vi "HeatFlow Log Data.vi"(9 "Log Stream":T2, 10 "HeatFlow Res Cfg":T1, 11 "tdms file":refnum<k34>) -> (0 "error out":errorcluster, 2 "Acquisition Stopped?":bool)   [LabVIEW 2019, in "Logging.lvlib"]
doc: "This VI uses the TDMS Write function to write data to a TDMS file."
uses:
  Logging.lvlib
  <extravilib>/ChannelInstances/Stream-var/)Channel.ctl
  HeatFlow Res Cfg.ctl
  HeatFlow Results States.ctl
  Acquisition/HeatFlow/HeatFlow Acq Data.ctl
  <extravilib>/ChannelInstances/Stream-var/Read With Abort.vi
  <extravilib>/ChannelInstances/Stream-var/EndpointRead.vi
  <extravilib>/ChannelInstances/Stream-var/)Channel.vi
  <resource>/ChannelSupport/_ChannelSupport/WaitIfNeeded.vi
  Acquisition/Acquisition.lvlib
  <extravilib>/ChannelInstances/Stream-var.lvlib
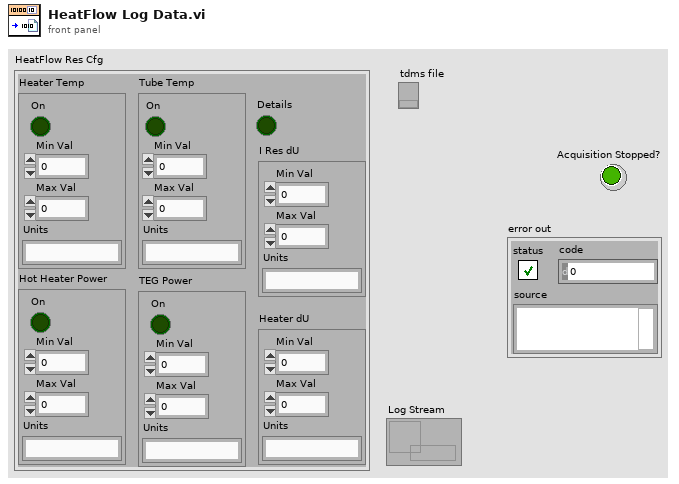
[diagram p1: front panel]
types:
  T1 = typedef "Logging.lvlib/HeatFlow Res Cfg.ctl" = cluster{"Heater Temp":cluster{"On":bool, "Min Val":dbl, "Max Val":dbl, "Units":string}, "Tube Temp":cluster{"On":bool, "Min Val":dbl, "Max Val":dbl, "Units":string}, "Hot Heater Power":cluster{"On":bool, "Min Val":dbl, "Max Val":dbl, "Units":string}, "TEG Power":cluster{"On":bool, "Min Val":dbl, "Max Val":dbl, "Units":string}, "Details":bool, "Heater dU":cluster{"Min Val":dbl, "Max Val":dbl, "Units":string}, "I Res dU":cluster{"Min Val":dbl, "Max Val":dbl, "Units":string}}
  T2 = typedef "Stream-var.lvlib/)Channel.ctl" = refnum<queue>
  T3 = typedef "Acquisition.lvlib/HeatFlow Acq Data.ctl" = cluster{"Time Stamp":timestamp, "Time Delta":u32, "LakeShore_Temp":cluster{"Tube_T_1":dbl, "Tube_T_2":dbl, "Tube_T_3":dbl, "Tube_T_4":dbl, "Tube_T_5":dbl, "Tube_T_6":dbl, "Tube_T_7":dbl, "Tube_T_8":dbl}, "Heaters":cluster{"I_Res_dU":dbl, "Heater_dU":dbl, "Hot_Side_I":dbl, "Hot_Side_P":dbl, "Cold_Ctrl_U":dbl, "Hot_Ctrl_U":dbl, "Hot_Side_T":dbl, "Cold_Side_T":dbl}, "TEG":cluster{"TEG_Load_dU":dbl, "TEG_Load_R":dbl, "TEG_Load_I":dbl, "TEG_Load_P":dbl, "TEG_eta":dbl, "TEG_dT":dbl, "TEG_U_open":dbl, "TEG_U_Test":dbl, "TEG_R_Test":dbl, "TEG_Rw":dbl}, "LastElement?":bool}
  T4 = typedef "Logging.lvlib/HeatFlow Results States.ctl" = enum16{"Start", "Timestamp", "Heater Temp", "Tube Temp", "Heater Power", "TEG Power", "Details", "End"}
  T5 = cluster{"Tube_T_1":dbl, "Tube_T_2":dbl, "Tube_T_3":dbl, "Tube_T_4":dbl, "Tube_T_5":dbl, "Tube_T_6":dbl, "Tube_T_7":dbl, "Tube_T_8":dbl}
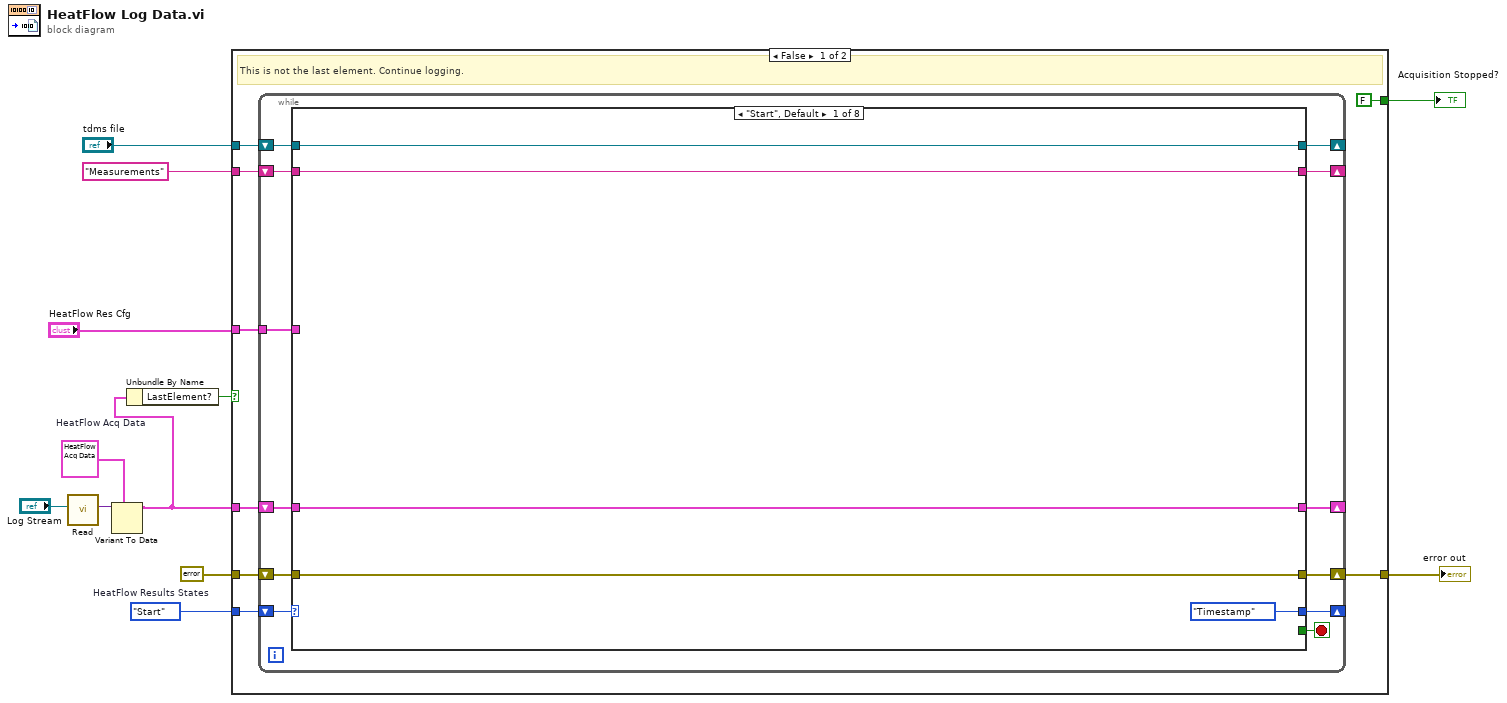
[diagram p0: block diagram]
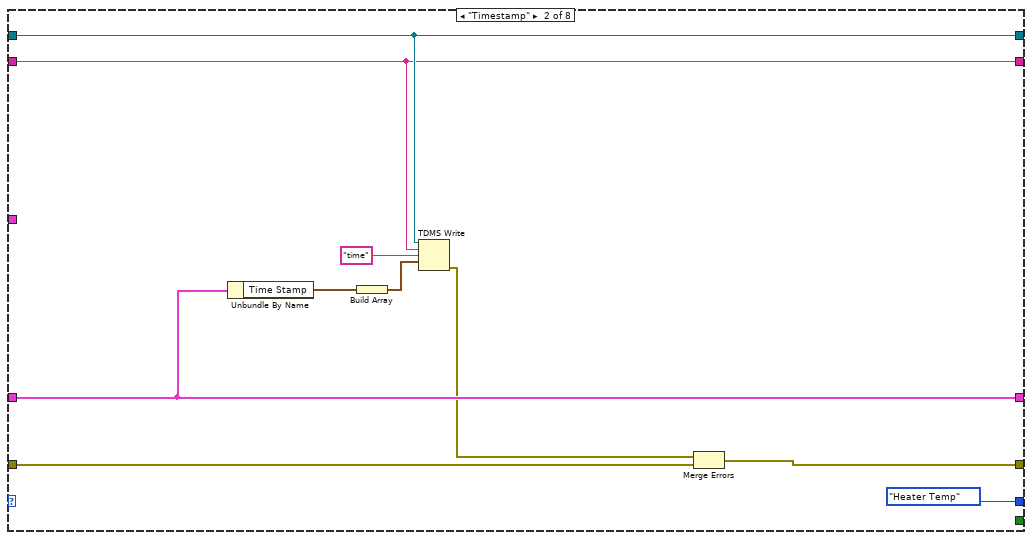
[diagram p2: hidden frame]
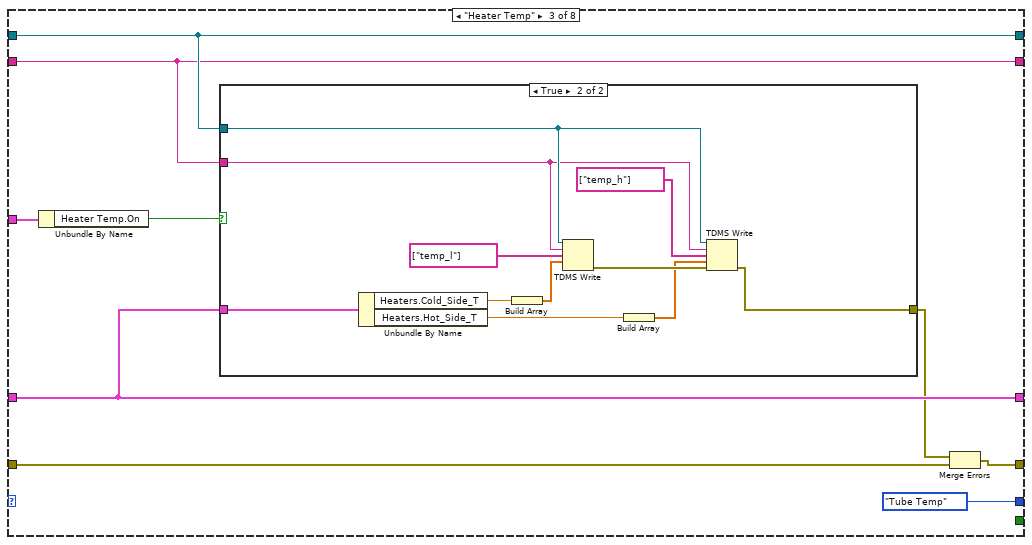
[diagram p3: hidden frame]
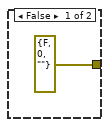
[diagram p4: hidden frame]
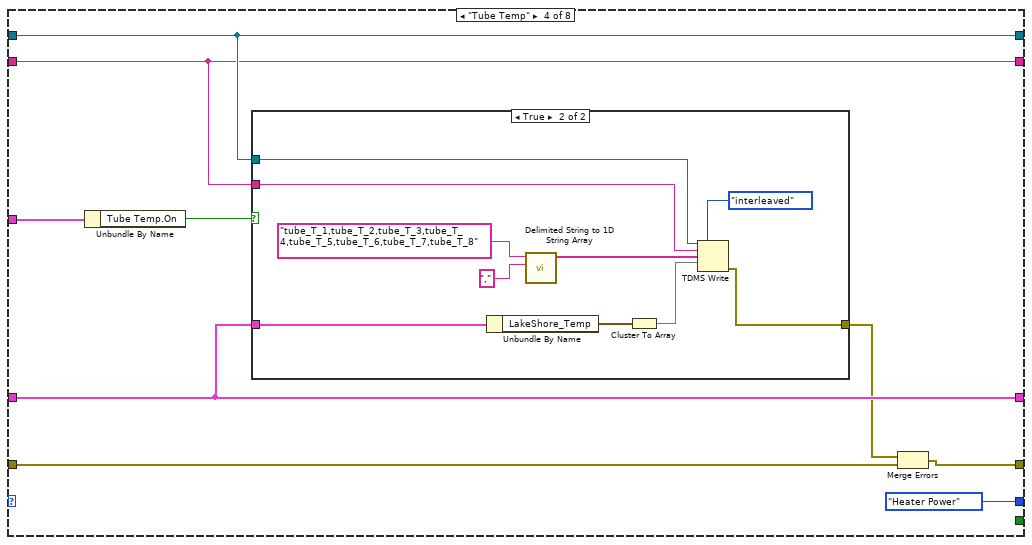
[diagram p5: hidden frame]
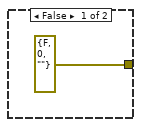
[diagram p6: hidden frame]
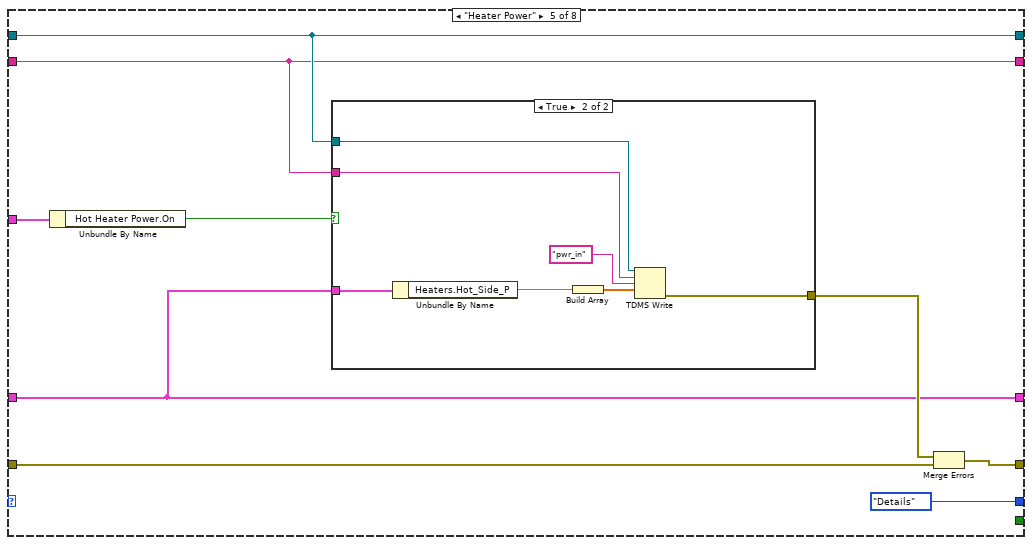
[diagram p7: hidden frame]
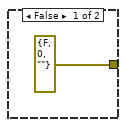
[diagram p8: hidden frame]
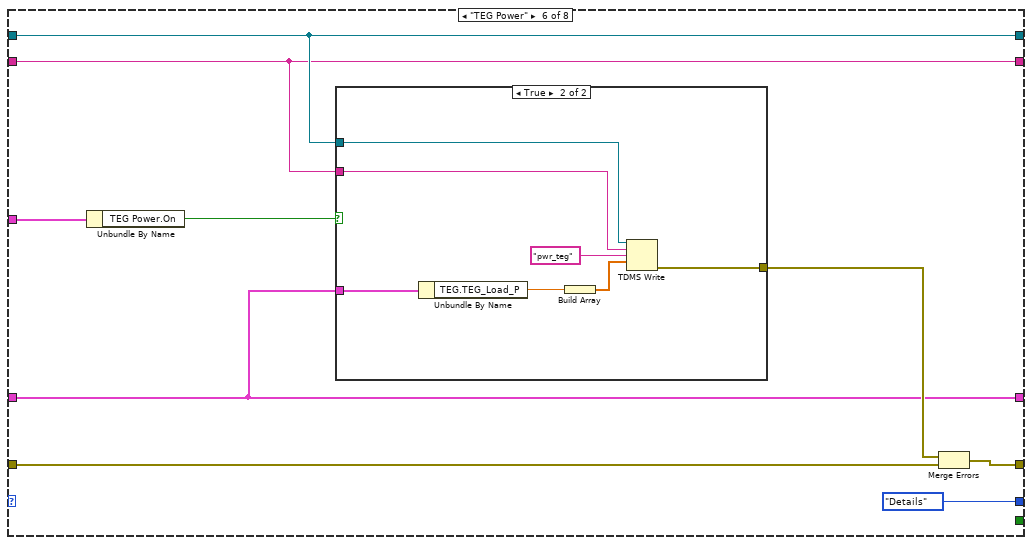
[diagram p9: hidden frame]
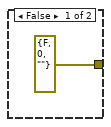
[diagram p10: hidden frame]
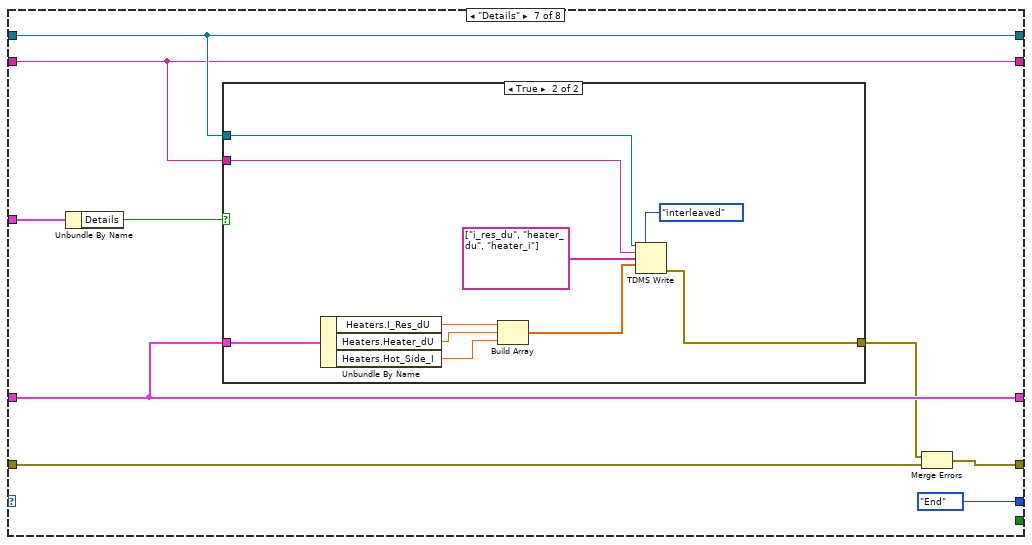
[diagram p11: hidden frame]
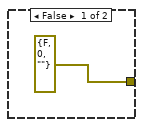
[diagram p12: hidden frame]
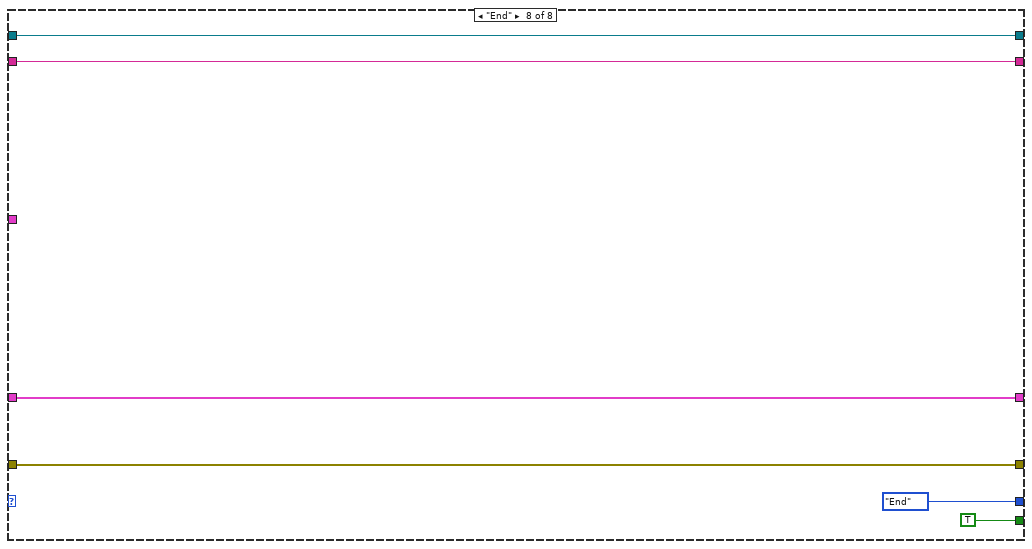
[diagram p13: hidden frame]
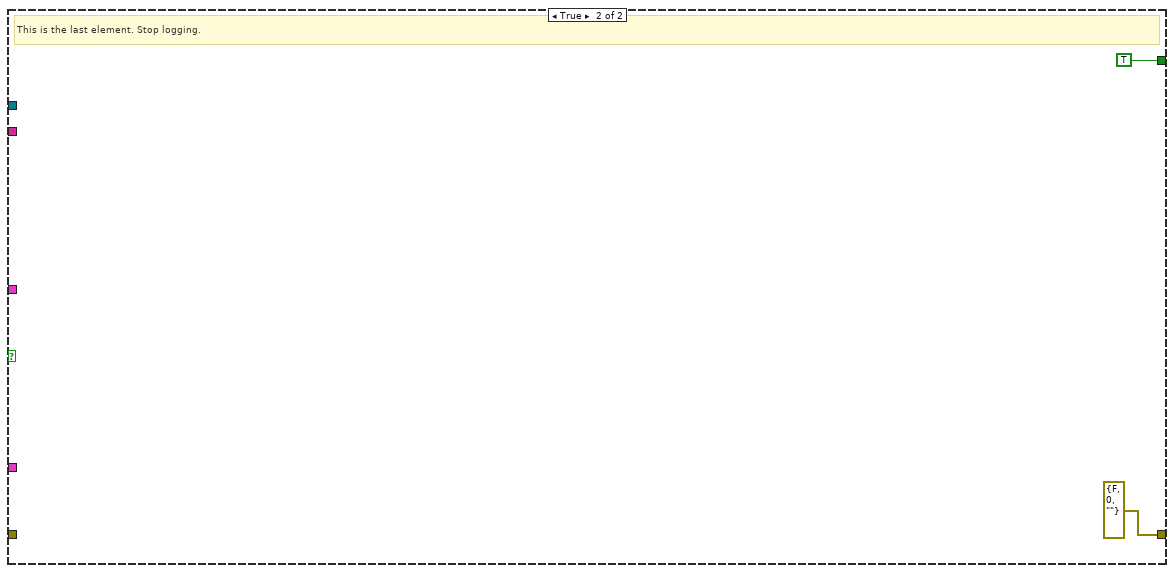
[diagram p14: hidden frame]
diagram:
  w3 = T3 {"Time Stamp"=timestamp(0 s since 1904-01-01), "Time Delta"=0, "LakeShore_Temp"={"Tube_T_1"=0.0, "Tube_T_2"=0.0, "Tube_T_3"=0.0, "Tube_T_4"=0.0, "Tube_T_5"=0.0, "Tube_T_6"=0.0, "Tube_T_7"=0.0, "Tube_T_8"=0.0}, "Heaters"={"I_Res_dU"=0.0, "Heater_dU"=0.0, "Hot_Side_I"=0.0, "Hot_Side_P"=0.0, "Cold_Ctrl_U"=0.0, "Hot_Ctrl_U"=0.0, "Hot_Side_T"=0.0, "Cold_Side_T"=0.0}, "TEG"={"TEG_Load_dU"=0.0, "TEG_Load_R"=0.0, "TEG_Load_I"=0.0, "TEG_Load_P"=0.0, "TEG_eta"=0.0, "TEG_dT"=0.0, "TEG_U_open"=0.0, "TEG_U_Test"=0.0, "TEG_R_Test"=0.0, "TEG_Rw"=0.0}, "LastElement?"=FALSE}  # HeatFlow Acq Data
  w7 = HeatFlow_Results_States."Start"  # HeatFlow Results States
  n1 = call <extravilib>:"Read.vi"("channel"="Log Stream") -> ("element"=w4:variant)  [unwired: 6 in, 4 out]
  n2 = Variant To Data(type=w3, Variant=w4) -> (data=w2:T3)  [unwired: 1 in, 1 out]
  n3 = Unbundle By Name(w2) -> ("LastElement?"=w6:bool)
  n4 = case shown="False" w6 {
    tunnel: [FALSE ("Acquisition Stopped?") TRUE ("Acquisition Stopped?")] -> w12
    tunnel: [w19 errorcluster {"status"=FALSE, "code"=0, "source"=""} ("error out")] -> w11
    tunnel: w7 -> [w18 _]
    tunnel: errorcluster {"status"=FALSE, "code"=0, "source"=""} ("error out") -> [w17 _]
    tunnel: "tdms file" -> [w16 _]
    tunnel: w2 -> [w15 _]
    tunnel: "Measurements" ("group name in (Untitled)") -> [w14 _]
    tunnel: "HeatFlow Res Cfg" -> [w13 _]
    frame False {
      # "This is not the last element. Continue logging."
      n5 = while {
        shift-right: [w32] -> _
        shift-left: w18 -> [w22]
        shift-right: [w28] -> _
        shift-left: w16 -> [w31]
        shift-right: [w29] -> w19
        shift-left: w17 -> [w30]
        shift-right: [w26] -> _
        shift-left: w15 -> [w27]
        shift-right: [w24] -> _
        shift-left: w14 -> [w25]
        tunnel: w13 -> [w21]
        stop <- w23 stop-if-true
        n6 = case shown="\"Start\", Default" w22 {
          tunnel: [HeatFlow_Results_States."Timestamp" ("Results") HeatFlow_Results_States."Heater Temp" ("Results") HeatFlow_Results_States."Tube Temp" ("Results") HeatFlow_Results_States."Heater Power" ("Results") HeatFlow_Results_States."Details" ("Results") HeatFlow_Results_States."Details" ("Results") HeatFlow_Results_States."End" ("Results") HeatFlow_Results_States."End" ("Results")] -> w32
          tunnel: w31 -> [w36 w44 w53 w75 w96 w113 w127 w148]
          tunnel: w30 -> [w33 w47 w50 w77 w97 w114 w130 w143]
          tunnel: [w33 w40 w49 w76 w94 w111 w124 w143] -> w29
          tunnel: [w36 w44 w53 w75 w96 w113 w127 w148] -> w28
          tunnel: w27 -> [w34 w43 w51 w74 w91 w108 w125 w145]
          tunnel: [w34 w43 w51 w74 w91 w108 w125 w145] -> w26
          tunnel: w25 -> [w35 w41 w52 w73 w95 w112 w126 w147]
          tunnel: [w35 w41 w52 w73 w95 w112 w126 w147] -> w24
          tunnel: [_ _ _ _ _ _ _ TRUE] -> w23
          tunnel: w21 -> [_ _ w55 w70 w90 w107 w129 _]
          frame "Start", Default {
          }
          frame "Timestamp" {
            n7 = Unbundle By Name(w43) -> ("Time Stamp"=w42:timestamp)
            n8 = Build Array(w42) -> (w46:timestamp[])
            n9 = TDMS Write(0:w44, 5:w41, 7:"time" ("group name in (Untitled)"), 9:w46) -> (15:w39:errorcluster)  [unwired: 2 in, 3 out]
            n10 = Merge Errors(w39, w47) -> (w40:errorcluster)
          }
          frame "Heater Temp" {
            n11 = Unbundle By Name(w55) -> ("Heater Temp.On"=w54:bool)
            n12 = case shown="True" w54 {
              tunnel: w51 -> [_ w68]
              tunnel: w53 -> [_ w60]
              tunnel: w52 -> [_ w59]
              tunnel: [errorcluster {"status"=FALSE, "code"=0, "source"=""} ("error constant") w58] -> w48
              frame False {
              }
              frame True {
                n13 = Unbundle By Name(w68) -> ("Heaters.Cold_Side_T"=w66:dbl, "Heaters.Hot_Side_T"=w61:dbl)
                n14 = Build Array(w66) -> (w65:dbl[])
                n15 = TDMS Write(0:w60, 5:w59, 7:string[] ["temp_l"] ("channel name(s) in (Untitled)"), 9:w65) -> (15:w64:errorcluster)  [unwired: 2 in, 3 out]
                n16 = Build Array(w61) -> (w62:dbl[])
                n17 = TDMS Write(0:w60, 5:w59, 7:string[] ["temp_h"] ("channel name(s) in (Untitled)"), 9:w62, 11:w64) -> (15:w58:errorcluster)  [unwired: 1 in, 3 out]
              }
            }
            n18 = Merge Errors(w48, w50) -> (w49:errorcluster)
          }
          frame "Tube Temp" {
            n19 = Unbundle By Name(w70) -> ("Tube Temp.On"=w69:bool)
            n20 = case shown="True" w69 {
              tunnel: w75 -> [_ w88]
              tunnel: w74 -> [_ w87]
              tunnel: w73 -> [_ w86]
              tunnel: [errorcluster {"status"=FALSE, "code"=0, "source"=""} ("error constant") w85] -> w71
              frame False {
              }
              frame True {
                n21 = Unbundle By Name(w87) -> ("LakeShore_Temp"=w84:T5)
                n22 = call <vilib>:"Delimited String to 1D String Array.vi"("delimiter"=",", "delimited string"="tube_T_1,tube_T_2,tube_T_3,tube_T_4,tube_T_5,tube_T_6,tube_T_7,tube_T_8" ("name to assign")) -> ("string array"=w81:string[])  [unwired: 9 in]
                n23 = Cluster To Array(cluster=w84) -> (array=w80:dbl[])
                n24 = TDMS Write(0:w88, 1:enum16{"decimated", "interleaved"}."interleaved" ("data layout (0:decimated)"), 5:w86, 7:w81, 9:w80) -> (15:w85:errorcluster)  [unwired: 1 in, 3 out]
              }
            }
            n25 = Merge Errors(w71, w77) -> (w76:errorcluster)
          }
          frame "Heater Power" {
            n26 = Unbundle By Name(w90) -> ("Hot Heater Power.On"=w89:bool)
            n27 = case shown="True" w89 {
              tunnel: w96 -> [_ w103]
              tunnel: w95 -> [_ w102]
              tunnel: [errorcluster {"status"=FALSE, "code"=0, "source"=""} ("error constant") w101] -> w93
              tunnel: w91 -> [_ w100]
              frame False {
              }
              frame True {
                n28 = Unbundle By Name(w100) -> ("Heaters.Hot_Side_P"=w99:dbl)
                n29 = Build Array(w99) -> (w105:dbl[])
                n30 = TDMS Write(0:w103, 5:w102, 7:"pwr_in" ("group name in (Untitled)"), 9:w105) -> (15:w101:errorcluster)  [unwired: 2 in, 3 out]
              }
            }
            n31 = Merge Errors(w93, w97) -> (w94:errorcluster)
          }
          frame "TEG Power" {
            n32 = Unbundle By Name(w107) -> ("TEG Power.On"=w106:bool)
            n33 = case shown="True" w106 {
              tunnel: w113 -> [_ w120]
              tunnel: w112 -> [_ w119]
              tunnel: [errorcluster {"status"=FALSE, "code"=0, "source"=""} ("error constant") w118] -> w110
              tunnel: w108 -> [_ w117]
              frame False {
              }
              frame True {
                n34 = Unbundle By Name(w117) -> ("TEG.TEG_Load_P"=w116:dbl)
                n35 = Build Array(w116) -> (w122:dbl[])
                n36 = TDMS Write(0:w120, 5:w119, 7:"pwr_teg" ("group name in (Untitled)"), 9:w122) -> (15:w118:errorcluster)  [unwired: 2 in, 3 out]
              }
            }
            n37 = Merge Errors(w110, w114) -> (w111:errorcluster)
          }
          frame "Details" {
            n38 = Unbundle By Name(w129) -> ("Details"=w128:bool)
            n39 = case shown="True" w128 {
              tunnel: w127 -> [_ w139]
              tunnel: w126 -> [_ w138]
              tunnel: w125 -> [_ w142]
              tunnel: [errorcluster {"status"=FALSE, "code"=0, "source"=""} ("error constant") w140] -> w123
              frame False {
              }
              frame True {
                n40 = Unbundle By Name(w142) -> ("Heaters.I_Res_dU"=w137:dbl, "Heaters.Heater_dU"=w136:dbl, "Heaters.Hot_Side_I"=w135:dbl)
                n41 = Build Array(w137, w136, w135) -> (w134:dbl[])
                n42 = TDMS Write(0:w139, 1:enum16{"decimated", "interleaved"}."interleaved" ("data layout (0:decimated)"), 5:w138, 7:string[] ["i_res_du", "heater_du", "heater_i"] ("channel name(s) in (Untitled)"), 9:w134) -> (15:w140:errorcluster)  [unwired: 1 in, 3 out]
              }
            }
            n43 = Merge Errors(w123, w130) -> (w124:errorcluster)
          }
          frame "End" {
          }
        }
      }
    }
    frame True {
      # "This is the last element. Stop logging."
    }
  }
  "error out" <- w11
  "Acquisition Stopped?" <- w12
